vi "Receive Value Change Msg.vi"(8 "error in (no error)":errorcluster, 10 "ValueChangeMsg":refnum<class "ValueChangeMsg.lvclass">, 11 "IViewable In":refnum<class "IViewable.lvclass">) -> (0 "error out":errorcluster, 3 "IViewable Out":refnum<class "IViewable.lvclass">)   [LabVIEW 2015, in "IViewable.lvlib" / "IViewable.lvclass"]
doc: "<License>\nCopyright © 2017 Composed Systems, LLC | All rights reserved\nwww.composed.io\n\nAuthor: Ethan Stern <ethan.stern@composed.io>\n\nThis software is provided \"AS IS\" WITHOUT WARRANTIES, either express or implied, AND IS FOR EDUCATIONAL PURPOSES ONLY.\n</License>"
uses:
  IViewable.lvclass
  AutoRegistration/ActorAutoRegistration Messages/ValueChangeMsg/ValueChangeMsg.lvclass
  <vilib>/ActorFramework/Actor/Actor.lvclass/Actor.ctl
  <vilib>/ActorFramework/Actor/Actor.lvclass
  AutoRegistration/ActorAutoRegistration Messages/EventDataMessage/EventDataMessage.lvclass
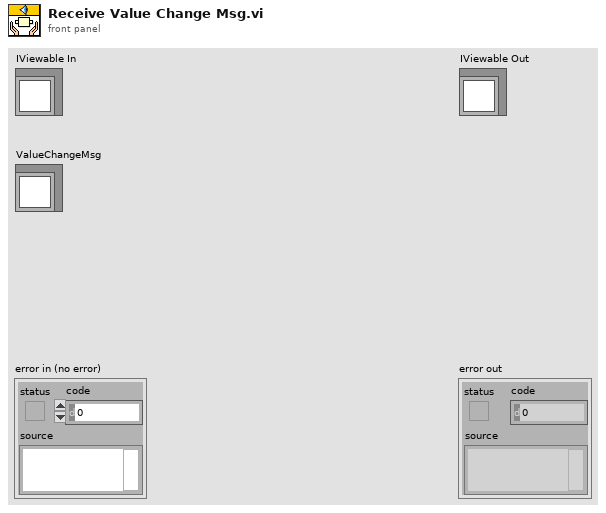
[diagram p1: front panel]
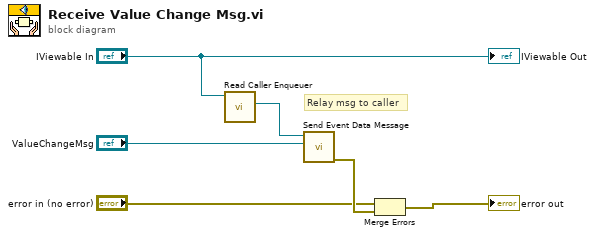
[diagram p0: block diagram]
diagram:
  # "Relay msg to caller"
  n1 = call <vilib>:"Read Caller Enqueuer.vi"("Actor"="IViewable In") -> ("Caller Enqueuer"=w5:refnum<class "Message Enqueuer.lvclass">)  [unwired: 10 in]
  n2 = call "Send Event Data Message.vi"("EventDataMessage in"="ValueChangeMsg", "Message Enqueuer in"=w5) -> ("error out"=w6:errorcluster)  [unwired: 9 in]
  n3 = Merge Errors("error in (no error)", w6) -> (→"error out":errorcluster)
  "IViewable Out" <- "IViewable In"
